vi "ma_SML Linear Weighting (real input).vi"(3 "reset?":bool, 4 "settings":T1, 5 "x":dbl[](array[numeric]) format="%.2f") -> (0 "data ready?":bool, 1 "averaged sofar":dbl format="%.2f", 2 "y":dbl[](array[numeric]) format="%.2f")   [LabVIEW 2020, in "NI_MAPro.lvlib"]
uses:
  NI_MAPro.lvlib
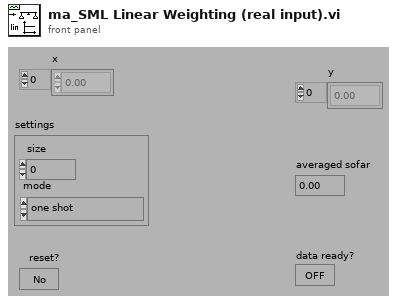
[diagram p1: front panel]
types:
  T1 = cluster{"size":dbl, "mode":enum16{"one shot", "auto restart one shot", "moving average", "continuous"}}
  T2 = enum16{"one shot", "auto restart one shot", "moving average", "continuous"}
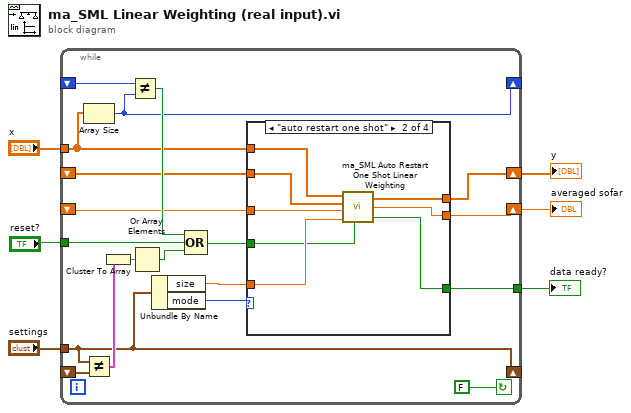
[diagram p0: block diagram]
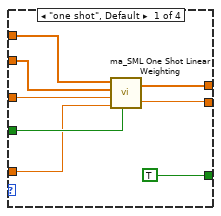
[diagram p2: hidden frame]
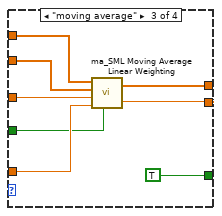
[diagram p3: hidden frame]
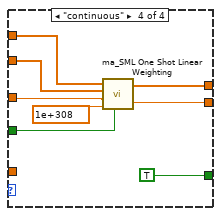
[diagram p4: hidden frame]
diagram:
  n1 = while {
    tunnel: [w8] -> w2
    tunnel: "x" -> [w11]
    shift-left: _ -> [w20]
    shift-right: [w19] -> _
    tunnel: "settings" -> [w17]
    shift-left: _ -> [w18]
    shift-right: [w17] -> _
    shift-left: _ -> [w13]
    shift-right: [w9] -> w1
    shift-left: _ -> [w12]
    shift-right: [w10] -> w3
    tunnel: "reset?" -> [w24]
    stop <- FALSE continue-if-true
    n2 = Array Size(array=w11) -> (size(s)=w19:i32)
    n3 = Not Equal?(x=w17, y=w18) -> (x != y?=w25:cluster{"size":bool, "mode":bool})
    n4 = Cluster To Array(cluster=w25) -> (array=w22:bool[])
    n5 = Not Equal?(x=w20, y=w19) -> (x != y?=w21:bool)
    n6 = Or Array Elements(Boolean array=w22) -> (logical OR=w23:bool)
    n7 = Unbundle By Name(w17) -> ("size"=w14:dbl, "mode"=w16:T2)
    n8 = Compound Arithmetic op=OR(w21, w24, w23) -> (w15:bool)
    n9 = case shown="\"auto restart one shot\"" w16 {
      tunnel: w15 -> [w33 w35 w46 w54]
      tunnel: w14 -> [w32 w36 w47 _]
      tunnel: w13 -> [w26 w37 w42 w50]
      tunnel: w12 -> [w31 w38 w48 w56]
      tunnel: w11 -> [w30 w39 w49 w57]
      tunnel: [w29 w41 w45 w53] -> w10
      tunnel: [w28 w40 w44 w52] -> w9
      tunnel: [TRUE ("DataReady") w34 TRUE ("DataReady") TRUE ("DataReady")] -> w8
      frame "one shot", Default {
        n10 = call "ma_SML One Shot Linear Weighting.vi"("x(n)"=w30, "y(n-1)"=w31, "averaged sofar(n-1)"=w26, "average size"=w32, "reset?"=w33) -> ("y(n)"=w29:dbl[], "averaged sofar(n)"=w28:dbl)
      }
      frame "auto restart one shot" {
        n11 = call "ma_SML Auto Restart One Shot Linear Weighting.vi"("x(n)"=w39, "y(n-1)"=w38, "averaged sofar(n-1)"=w37, "average size"=w36, "reset?"=w35) -> ("y(n)"=w41:dbl[], "averaged sofar(n)"=w40:dbl, "data ready?"=w34:bool)
      }
      frame "moving average" {
        n12 = call "ma_SML Moving Average Linear Weighting.vi"("x(n)"=w49, "y(n-1)"=w48, "averaged sofar(n-1)"=w42, "average size"=w47, "reset?"=w46) -> ("y(n)"=w45:dbl[], "averaged sofar(n)"=w44:dbl)
      }
      frame "continuous" {
        n13 = call "ma_SML One Shot Linear Weighting.vi"("x(n)"=w57, "y(n-1)"=w56, "averaged sofar(n-1)"=w50, "average size"=1e+308 ("Average Size"), "reset?"=w54) -> ("y(n)"=w53:dbl[], "averaged sofar(n)"=w52:dbl)
      }
    }
  }
  "averaged sofar" <- w1
  "y" <- w3
  "data ready?" <- w2
